vi "Set Create Merge Commit.vi"(8 "error in (no error)":errorcluster, 10 "no-ff":bool caption="Create Merge Commit (--no-ff)", 11 "No-Conflicts Merge in":refnum<class "No-Conflicts Merge.lvclass">) -> (0 "error out":errorcluster, 3 "No-Conflicts Merge out":refnum<class "No-Conflicts Merge.lvclass">)   [LabVIEW 2017, in "Git-LabVIEW.lvlib" / "No-Conflicts Merge.lvclass"]
uses:
  No-Conflicts Merge.lvclass
  No-Conflicts Merge.lvclass/No-Conflicts Merge.ctl
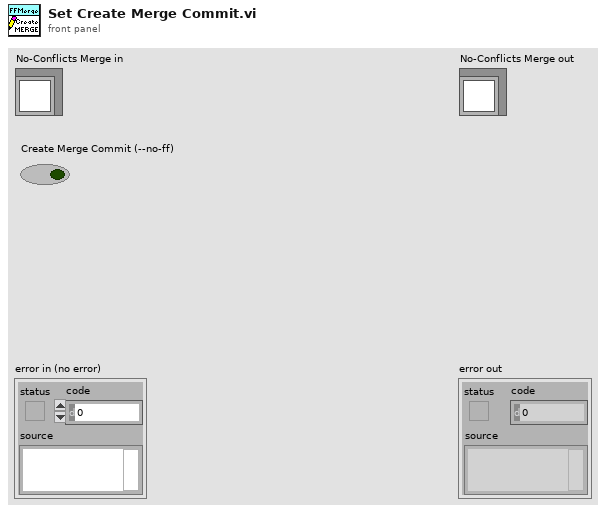
[diagram p1: front panel]
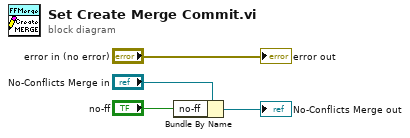
[diagram p0: block diagram]
diagram:
  n1 = Bundle By Name(cluster="No-Conflicts Merge in", "no-ff"="no-ff") -> (→"No-Conflicts Merge out":refnum<class "No-Conflicts Merge.lvclass">)
  "error out" <- "error in (no error)"
